vi "Auton Globals.vi"() -> ()   [LabVIEW 2012]
panel:
  in  "1: Alignment Acelleration":dbl
  in  "1: Alignment Threshold":dbl
  in  "1: Run Alignment":bool
  in  "4: Drive Stop Range":dbl=36.0
  in  "4: Drive Speed":dbl=0.225
  in  "4: Arm Lower Range":dbl=30.48
  in  "2: Stop Timer":dbl=1500.0
  in  "2: Y Speed":dbl=0.01
  in  "0: Drive Speed":dbl=0.25
  in  "0: Speed Throttle Dist":dbl=36.0
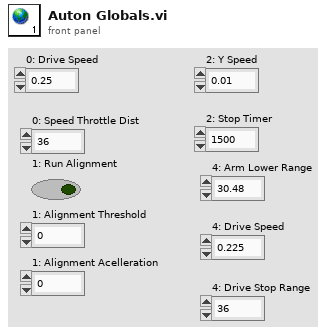
[diagram p1: front panel]
diagram:
